vi "programa7_CONDICIONES.vi"() -> ()   [LabVIEW 2013]
panel:
  out "ALARMA":bool
  out "Temperatura":dbl(slide) scale=0.0..100.0
  out "Velocidad S. RAPIDA":bool
  out "Velocidad RAPIDA":bool
  out "Velocidad lenta":bool
  out "Velocidad":i32(knob) scale=0.0..220.0
  # "SE TIENE QUE GENERAR LA VELOCIDAD ENTRE 1-220 \nLUEGO SE ENCIENDEN LOS LED DE ACUERDO A LA VELOCIDAD\n\n1-80 LENTA\n81-120 RAPIDA\n212-220 MUY RAPIDA\n\nLUEGO SI LA TEMPERATURA ESTA ARRIBA DE LOS 75 GRADOS Y LA VELOCIDAD\nES MUY RAPIDA SE TIENE QUE ENCENDER EL LED DE ALARMA"
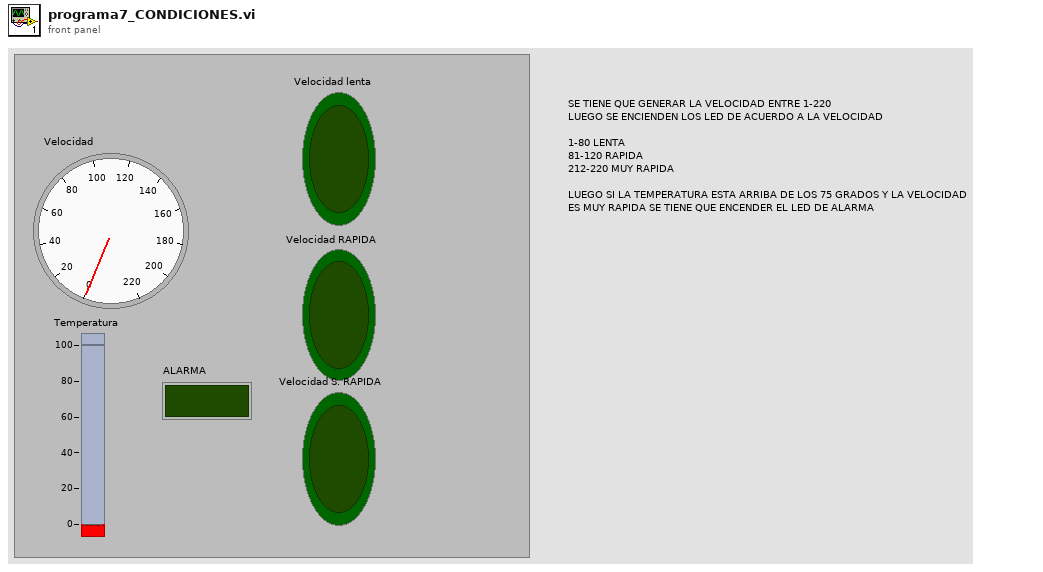
[diagram p1: front panel]
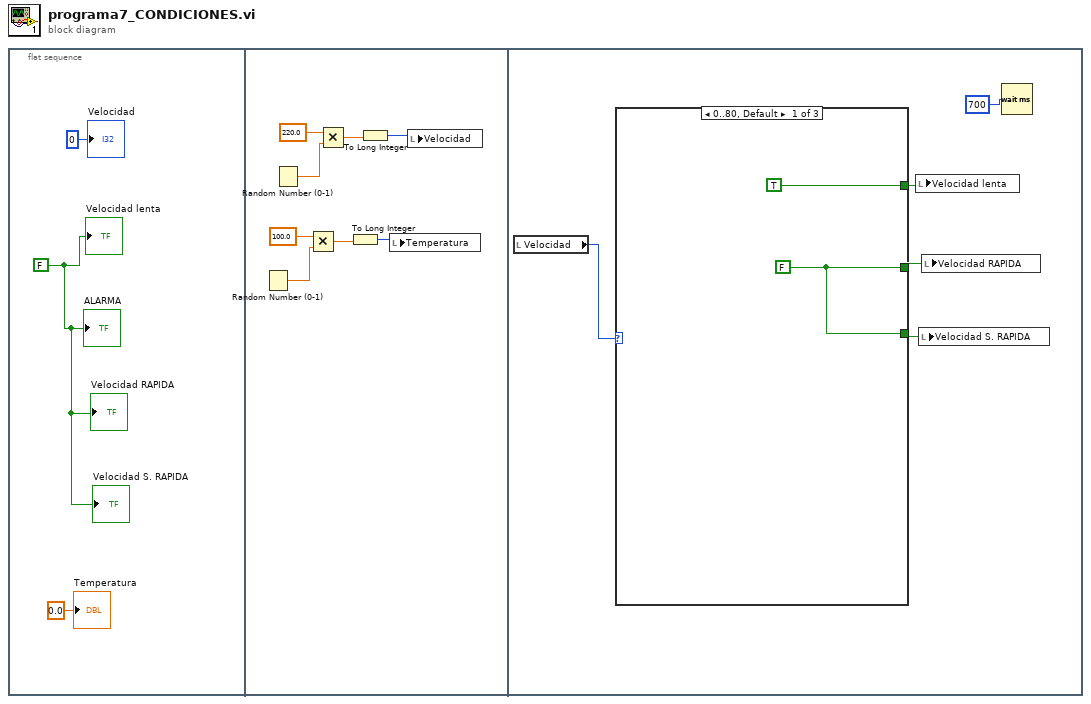
[diagram p0: block diagram]
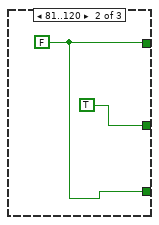
[diagram p2: hidden frame]
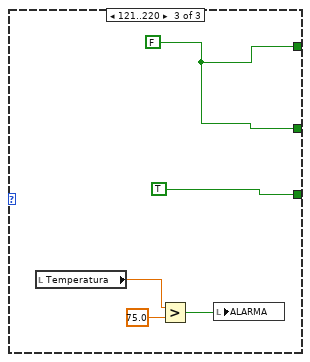
[diagram p3: hidden frame]
diagram:
  n1 = flat-sequence {
    frame #0 {
      w2 = FALSE
      "Velocidad" <- 0 ("Velocidad")
      "ALARMA" <- w2
      "Velocidad lenta" <- w2
      "Velocidad RAPIDA" <- w2
      "Velocidad S. RAPIDA" <- w2
      "Temperatura" <- 0.0 ("Temperatura")
    }
    frame #1 {
      n2 = Random Number (0-1)() -> (number: 0 to 1=w5:dbl)
      n3 = Random Number (0-1)() -> (number: 0 to 1=w10:dbl)
      n4 = Multiply(x=100.0, y=w5) -> (x*y=w6:dbl)
      n5 = Multiply(x=220.0, y=w10) -> (x*y=w9:dbl)
      n6 = To Long Integer(number=w6) -> (32bit integer=w7:i32)
      n7 = To Long Integer(number=w9) -> (32bit integer=w8:i32)
      n8 = local write "Temperatura"(w7) -> ()
      n9 = local write "Velocidad"(w8) -> ()
    }
    frame #2 {
      n10 = local read "Velocidad"() -> (w16:i32)
      n11 = case shown="0..80, Default" w16 {
        tunnel: [TRUE w20 w24] -> w15
        tunnel: [w17 TRUE w24] -> w14
        tunnel: [w17 w20 TRUE] -> w13
        frame 0..80, Default {
          w17 = FALSE
        }
        frame 81..120 {
          w20 = FALSE
        }
        frame 121..220 {
          w24 = FALSE
          n12 = local read "Temperatura"() -> (w21:dbl)
          n13 = Greater?(x=w21, y=75.0) -> (0:w23:bool)
          n14 = local write "ALARMA"(w23) -> ()
        }
      }
      n15 = local write "Velocidad lenta"(w15) -> ()
      n16 = local write "Velocidad S. RAPIDA"(w13) -> ()
      n17 = local write "Velocidad RAPIDA"(w14) -> ()
      n18 = Wait (ms)(milliseconds to wait=700) -> ()  [unwired: 1 out]
    }
  }
